vi "UriToImage.vi"(5 "image Path":path, 11 "error in (no error)":errorcluster) -> (6 ".NET object":refnum<k24>, 15 "error out":errorcluster)   [LabVIEW 2018, in "DataGridView.lvclass"]
uses:
  DataGridView.lvclass
  System.Drawing
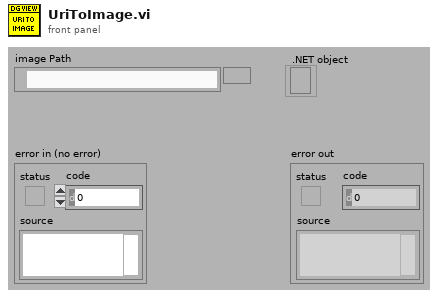
[diagram p1: front panel]
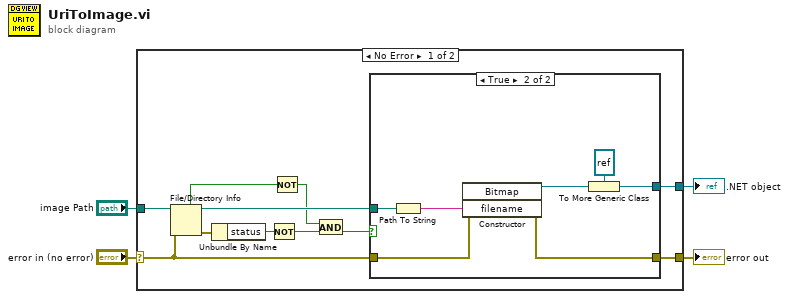
[diagram p0: block diagram]
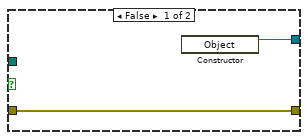
[diagram p2: hidden frame]
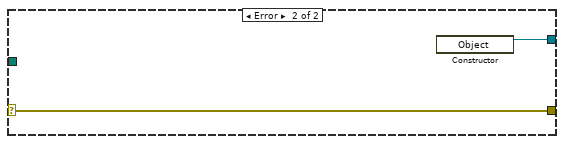
[diagram p3: hidden frame]
diagram:
  n1 = case shown="No Error" "error in (no error)" {
    selector: "error in (no error)" -> [w10 w26]
    tunnel: [w11 w26] -> w3
    tunnel: "image Path" -> [w13 _]
    tunnel: [w5 w25] -> w1
    frame No Error {
      n2 = File/Directory Info(path=w13, error in=w10) -> (path out=w9:path, directory=w7:bool, error out=w14:errorcluster)  [unwired: 4 out]
      n3 = Unbundle By Name(w14) -> ("status"=w15:bool)
      n4 = Not(x=w15) -> (.not. x?=w12:bool)
      n5 = Not(x=w7) -> (.not. x?=w6:bool)
      n6 = And(x=w6, y=w12) -> (x .and. y?=w8:bool)
      n7 = case shown="True" w8 {
        tunnel: w10 -> [w17 w22]
        tunnel: [w17 w18] -> w11
        tunnel: w9 -> [_ w24]
        tunnel: [w16 w19] -> w5
        frame False {
          n8 = constructor class="Object"() -> (reference out=w16:refnum<k24>)  [unwired: 3 in, 2 out]
        }
        frame True {
          n9 = Path To String(path=w24) -> (string=w23:string)
          n10 = constructor class="Bitmap"(error in=w22, "filename"=w23) -> (reference out=w20:refnum<k24>, error out=w18:errorcluster)  [unwired: 2 in, 2 out]
          n11 = To More Generic Class(target class=refnum<k24> refnum (".NET object"), reference=w20) -> (generic class reference=w19:refnum<k24>)
        }
      }
    }
    frame Error {
      n12 = constructor class="Object"() -> (reference out=w25:refnum<k24>)  [unwired: 3 in, 2 out]
    }
  }
  "error out" <- w3
  ".NET object" <- w1
